vi "Instrument.GetPrivateEvents.vi"(8 "error in (no error)":errorcluster, 11 "Instrument":refnum<class "Instrument.lvclass">) -> (0 "error out":errorcluster, 2 "Private Events":T1, 3 "Instrument out":refnum<class "Instrument.lvclass">)   [LabVIEW 2020, in "Instrument.lvclass"]
doc: "---------------------------------------------------------------\nJKI State Machine Objects™\nhttp://jki.net/state-machine-objects/\nCopyright (C) 2005-2015, JKI <info@jki.net>\nALL RIGHTS RESERVEDJKI State Machine Objects (SMO) 1.0.0.5\nJKI - JKI\nCopyright (c) 2016, JKI"
uses:
  Instrument.lvclass
  Typedefs/PrivateEvents--Cluster.ctl
  Typedefs/API Inputs--Cluster.ctl
  Typedefs/Data.ctl
  Instrument.lvclass/Instrument.ctl
panel:
  # "For instructions on how to use the JKI State Machine Objects, examples and video tutorials, visit:\nhttp://jki.net/state-machine-objects/\n\nJKI State Machine Objects™\nhttp://jki.net/state-machine-objects/\nCopyright (C) 2005-2015, JKI <info@jki.net>\nALL RIGHTS RESERVED"
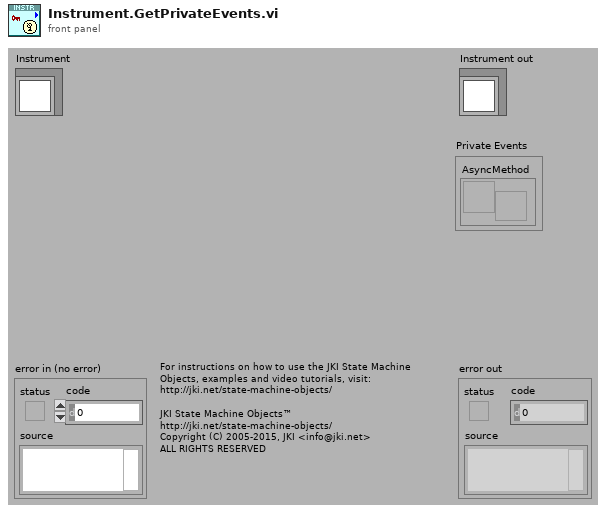
[diagram p1: front panel]
types:
  T1 = typedef "Instrument.lvclass/PrivateEvents--Cluster.ctl" = cluster{"AsyncMethod":refnum<user-event>}
  T2 = typedef "Instrument.lvclass/PrivateData--Ref.ctl" = refnum<data-value>
  T3 = typedef "Instrument.lvclass/PrivateData--Cluster.ctl" = cluster{"Configuration":T4, "Public Events":T5, "Protected Events":T6, "Private Events":T1, "Data":T7}
  T4 = typedef "Instrument.lvclass/Configuration--Cluster.ctl" = cluster{"Suffix":string}
  T5 = typedef "Instrument.lvclass/PublicEvents--Cluster.ctl" = cluster{"Data Changed":refnum<user-event>}
  T6 = typedef "Instrument.lvclass/ProtectedEvents--Cluster.ctl" = cluster{"API_Template":refnum<user-event>}
  T7 = typedef "Instrument.lvclass/Data.ctl" = string
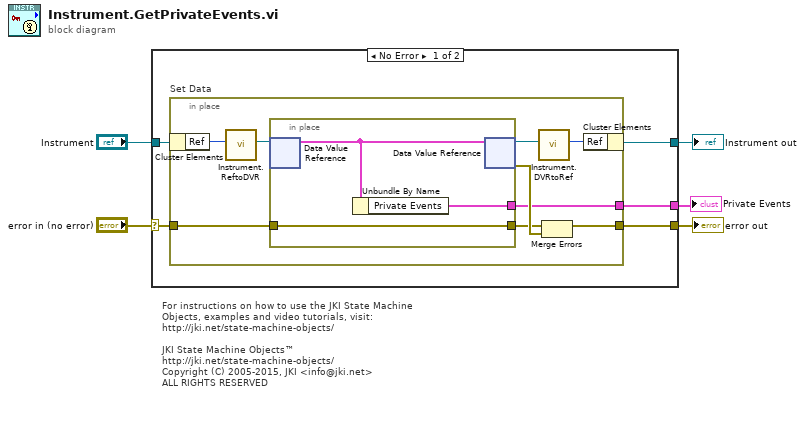
[diagram p0: block diagram]
diagram:
  # "For instructions on how to use the JKI State Machine Objects, examples and video tutorials, visit:\nhttp://jki.net/state-machine-objects/\n\nJKI State Machine Objects™\nhttp://jki.net/state-machine-objects/\nCopyright (C) 2005-2015, JKI <info@jki.net>\nALL RIGHTS RESERVED"
  n1 = case shown="No Error" "error in (no error)" {
    selector: "error in (no error)" -> [w9 w23]
    tunnel: "Instrument" -> [w10 w24]
    tunnel: [w8 w23] -> w4
    tunnel: [w7 w24] -> w3
    tunnel: [w6 _] -> w1
    frame No Error {
      n2 = in-place "Set Data" {
        in-place-border: w9 -> [w19]
        in-place-border: [w16] -> w8
        in-place-border: [w11] -> w6
        n3 = in-place-cluster #1(w10) -> ("Ref"=w15:u32)
        n4 = call "Instrument.ReftoDVR.vi"("Ref"=w15) -> ("Ref"=w14:T2)  [unwired: 10 in]
        n5 = in-place {
          in-place-border: w19 -> [w22]
          in-place-border: [w22] -> w17
          in-place-border: [w20] -> w11
          n6 = in-place-dvr #2(w14) -> (w21:T3)  [unwired: 1 out]
          n7 = Unbundle By Name(w21) -> ("Private Events"=w20:T1)
          n8 = in-place-dvr #2(w21) -> (w13:T2, w18:errorcluster)
        }
        n9 = call "Instrument.DVRtoRef.vi"("Ref"=w13) -> ("Ref"=w12:u32)  [unwired: 10 in]
        n10 = Merge Errors(w17, w18) -> (w16:errorcluster)
        n11 = in-place-cluster #1("Ref"=w12) -> (w7:refnum<class "Instrument.lvclass">)
      }
    }
    frame Error {
    }
  }
  "error out" <- w4
  "Instrument out" <- w3
  "Private Events" <- w1
